vi "LOGIN AUTHENTICATION.vi"(8 "error in":errorcluster, 11 "Credentials File Path":path) -> (0 "error out":errorcluster, 1 "USER EXISTS?":bool, 2 "user?":string)   [LabVIEW 2015]
panel:
  in  "hide(F)/show(T)":bool
  in  "OK":bool
  in  "Cancel":bool
  in  "Password":string="********"
  in  "User Name":string="Enter User Name Here"
  # "User Authentication"
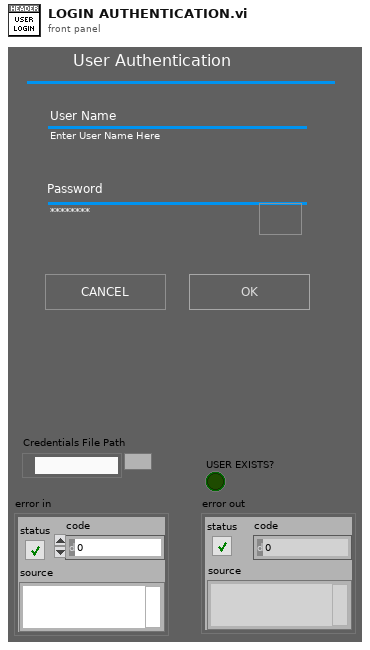
[diagram p1: front panel]
types:
  T1 = enum8{"Enabled", "Disabled", "Disabled and Grayed Out"}
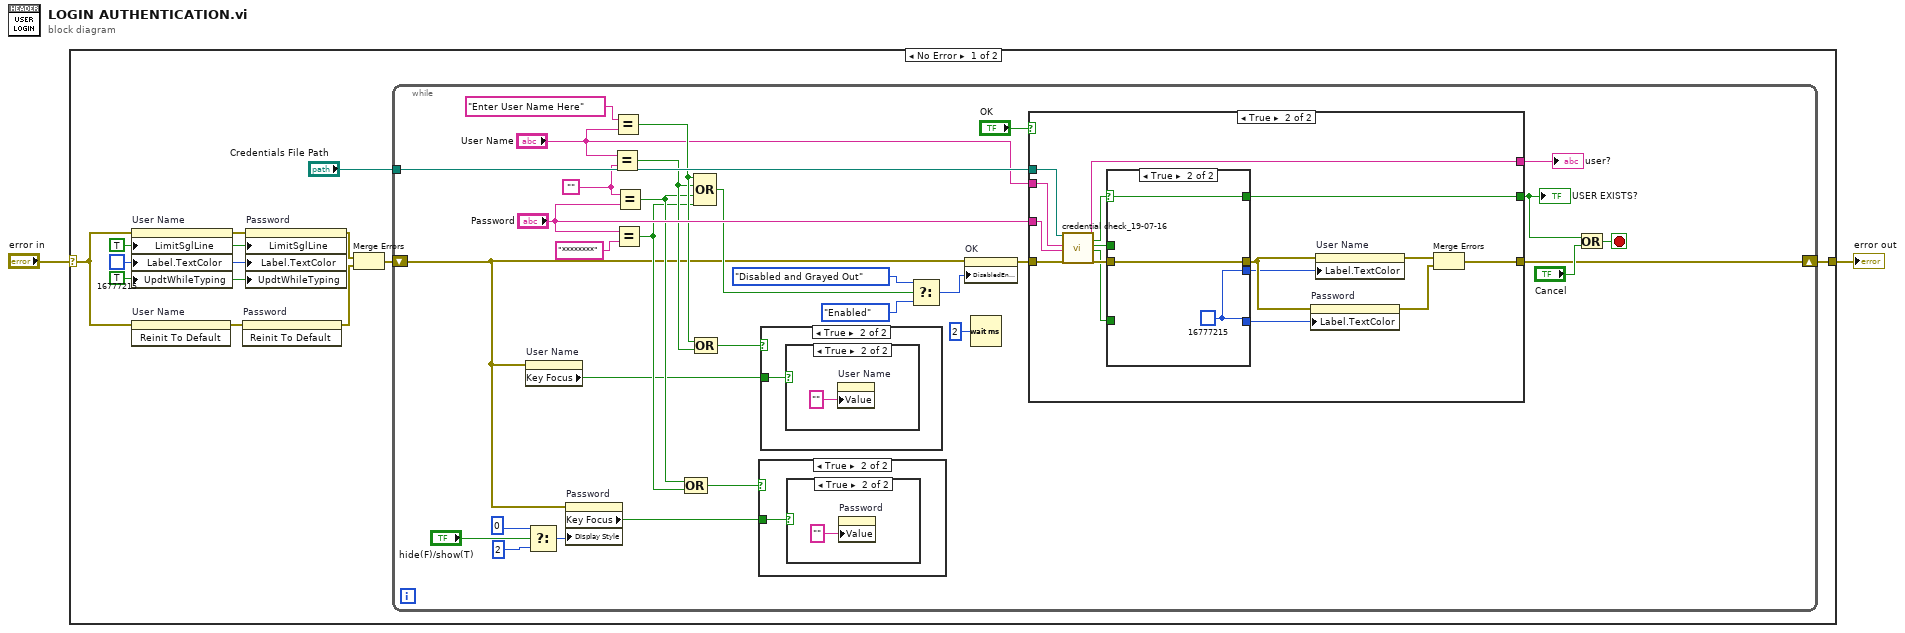
[diagram p0: block diagram]
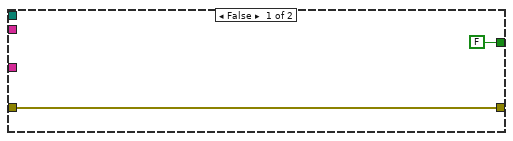
[diagram p6: hidden frame]
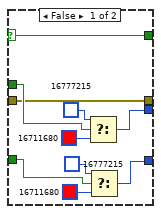
[diagram p7: hidden frame]
diagram:
  n1 = case shown="No Error" "error in" {
    selector: "error in" -> [w9 w80]
    tunnel: [w13 w80] -> w1
    frame No Error {
      w3 = TRUE ("Update While Typing?")
      w4 = u32 16777215
      w10 = TRUE
      n2 = property on="User Name" class="Str"(error in=w9, "LimitSglLine"=w10, "Label.TextColor"=w4, "UpdtWhileTyping"=w3) -> (error out=w11:errorcluster)  [unwired: 1 in, 1 out]
      n3 = invoke on="User Name" class="Str" method="Reinit To Default"(error in=w9) -> (error out=w12:errorcluster)  [unwired: 2 in, 2 out]
      n4 = invoke on="Password" class="Str" method="Reinit To Default"(error in=w12) -> (error out=w6:errorcluster)  [unwired: 2 in, 2 out]
      n5 = property on="Password" class="Str"(error in=w11, "LimitSglLine"=w10, "Label.TextColor"=w4, "UpdtWhileTyping"=w3) -> (error out=w7:errorcluster)  [unwired: 1 in, 1 out]
      n6 = Merge Errors(w7, w6) -> (w5:errorcluster)
      n7 = while {
        shift-right: [w17] -> w13
        shift-left: w5 -> [w19]
        tunnel: "Credentials File Path" -> [w40]
        stop <- w42 stop-if-true
        w37 = ""
        n8 = property on="User Name" class="Str"(error in=w19) -> ("Key Focus"=w25:bool)  [unwired: 1 in, 2 out]
        n9 = Select(t=u32 0, s="hide(F)/show(T)", f=u32 2 ("Display Style")) -> (s? t:f=w24:u32)
        n10 = property on="Password" class="Str"(error in=w19, "Display Style"=w24) -> ("Key Focus"=w26:bool)  [unwired: 1 in, 2 out]
        n11 = Equal?(x="User Name", y=w37) -> (x = y?=w29:bool)
        n12 = Equal?(x="Enter User Name Here", y="User Name") -> (x = y?=w30:bool)
        n13 = Equal?(x="Password", y="********") -> (x = y?=w27:bool)
        n14 = Equal?(x=w37, y="Password") -> (x = y?=w28:bool)
        n15 = Compound Arithmetic op=OR(w28, w27) -> (w15:bool)
        n16 = Compound Arithmetic op=OR(w30, w29, w28, w27) -> (w23:bool)
        n17 = Compound Arithmetic op=OR(w30, w29) -> (w16:bool)
        n18 = case shown="True" w15 {
          tunnel: w26 -> [_ w45]
          frame False {
          }
          frame True {
            n19 = case shown="True" w45 {
              frame False {
              }
              frame True {
                n20 = property on="Password" class="Str"("Value"="" ("User Name")) -> ()  [unwired: 2 in, 2 out]
              }
            }
          }
        }
        n21 = case shown="True" w16 {
          tunnel: w25 -> [_ w47]
          frame False {
          }
          frame True {
            n22 = case shown="True" w47 {
              frame False {
              }
              frame True {
                n23 = property on="User Name" class="Str"("Value"="" ("User Name")) -> ()  [unwired: 2 in, 2 out]
              }
            }
          }
        }
        n24 = Select(t=T1."Disabled and Grayed Out" ("Disabled"), s=w23, f=T1."Enabled" ("Disabled")) -> (s? t:f=w20:T1)
        n25 = property on="OK" class="Bool"(error in=w19, "DisabledEnum"=w20) -> (error out=w44:errorcluster)  [unwired: 1 in, 1 out]
        n26 = Wait (ms)(milliseconds to wait=u32 2) -> ()  [unwired: 1 out]
        n27 = case shown="True" "OK" {
          tunnel: "User Name" -> [_ w66]
          tunnel: "Password" -> [_ w65]
          tunnel: w44 -> [w50 w64]
          tunnel: [w50 w53] -> w17
          tunnel: [FALSE w61] -> w41
          tunnel: [_ w63] -> w43
          tunnel: w40 -> [_ w60]
          frame False {
          }
          frame True {
            n28 = call "credential check_19-07-16.vi"("Credentials file path"=w60, "USER NAME"=w66, "PASSWORD"=w65, "error in"=w64) -> ("user?"=w63:string, "USER EXISTS?"=w62:bool, "User Name"=w58:bool, "Password"=w57:bool, "error out"=w59:errorcluster)  [unwired: 11 in]
            n29 = case shown="True" w62 {
              selector: w62 -> [w76 w79]
              tunnel: [w76 w79] -> w61
              tunnel: w59 -> [w72 w77]
              tunnel: [w72 w77] -> w56
              tunnel: w58 -> [w75 _]
              tunnel: w57 -> [w68 _]
              tunnel: [w71 w78] -> w52
              tunnel: [w67 w78] -> w51
              frame False {
                n30 = Select(t=u32 16777215, s=w75, f=u32 16711680) -> (s? t:f=w71:u32)
                n31 = Select(t=u32 16777215, s=w68, f=u32 16711680) -> (s? t:f=w67:u32)
              }
              frame True {
                w78 = u32 16777215
              }
            }
            n32 = property on="Password" class="Str"(error in=w56, "Label.TextColor"=w51) -> (error out=w54:errorcluster)  [unwired: 1 in, 1 out]
            n33 = property on="User Name" class="Str"(error in=w56, "Label.TextColor"=w52) -> (error out=w55:errorcluster)  [unwired: 1 in, 1 out]
            n34 = Merge Errors(w55, w54) -> (w53:errorcluster)
          }
        }
        "USER EXISTS?" <- w41
        "user?" <- w43
        n35 = Or(x=w41, y="Cancel") -> (x .or. y?=w42:bool)
      }
    }
    frame Error {
    }
  }
  "error out" <- w1
